vi "MDM_test.vi"() -> ()   [LabVIEW 2014]
uses:
  sub_VI/Control 1.ctl
  controls/thrust_control.ctl
  controls/diag.ctl
  <vilib>/Instr/_visa.llb/VISA Configure Serial Port (Instr).vi
  <vilib>/Utility/inputDevices.llb/joystickAcquire.vi
panel:
  in  "Calibrate Pressure":sgl=15.0 format="%_3f"
  in  "Calibrate Pressure":bool
  out "Pressure":sgl(knob) scale=-100.0..100.0
  out "diag":T1 {"calibrate pressure" format="%_6f"}
  out "axis info":T2
  out "button info":T3
  out "direction info":T4
  in  "index":u16
  in  "Address 2":u16
  in  "Forward":bool
  in  "Thrust":u16
  in  "VISA resource name 2":refnum<visa-resource-name>
  in  "Read Diag":bool
  in  "Thruster 1":T5 {"Thrust" scale=0.0..100.0}
  in  "baud rate (9600)":T6=19200
  in  "stop":bool
  in  "Address":u16
  in  "VISA resource name":refnum<visa-resource-name>="COM5"
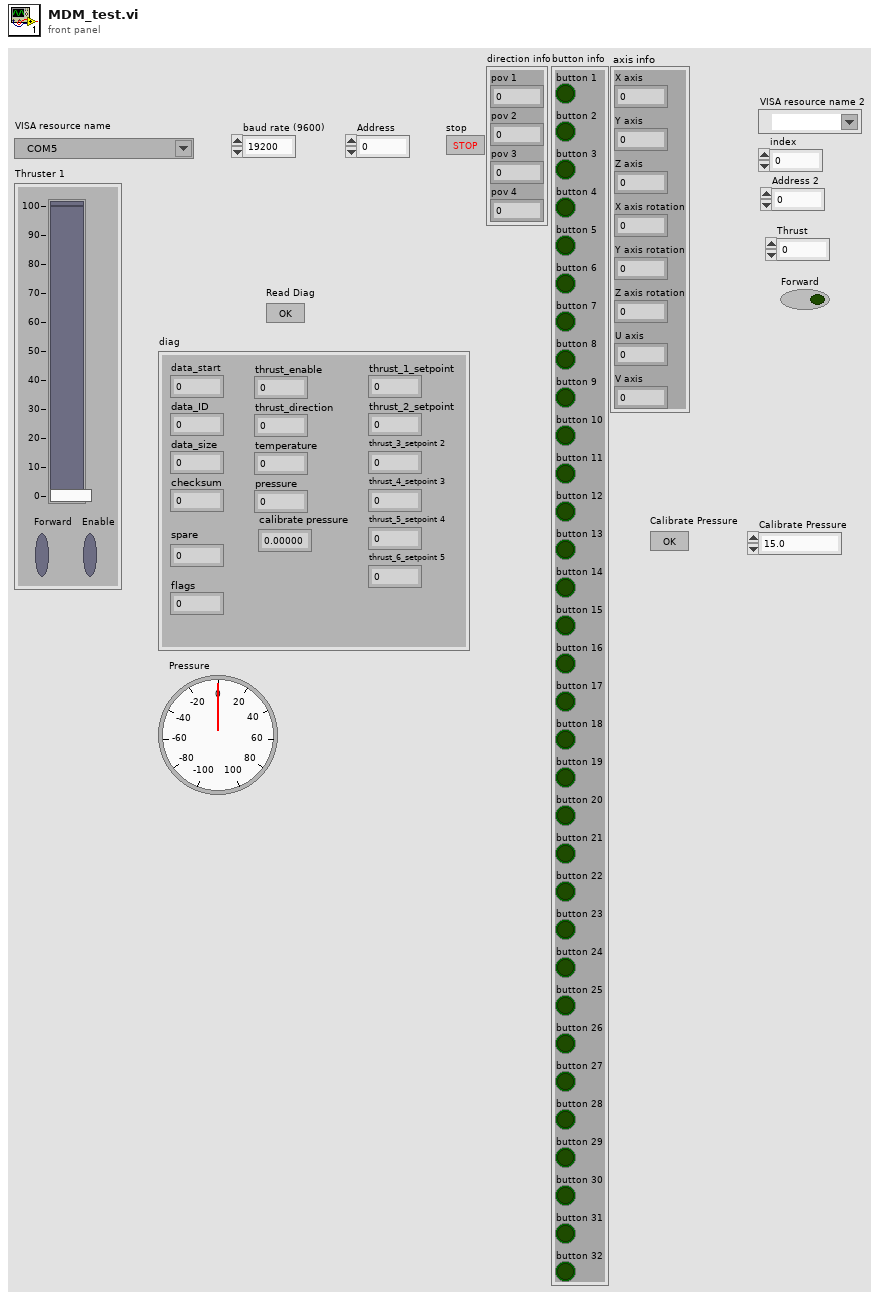
[diagram p1: front panel]
types:
  T1 = typedef "diag.ctl" = cluster{"data_start":u16, "data_ID":u16, "data_size":u16, "thrust_enable":u8, "thrust_direction":u8, "temperature":sgl, "pressure":sgl, "thrust_1_setpoint":u16, "thrust_2_setpoint":u16, "thrust_3_setpoint 2":u16, "thrust_4_setpoint 3":u16, "thrust_5_setpoint 4":u16, "thrust_6_setpoint 5":u16, "spare":u16, "flags":u16, "calibrate pressure":sgl, "checksum":u16}
  T2 = cluster{"X axis":i32, "Y axis":i32, "Z axis":i32, "X axis rotation":i32, "Y axis rotation":i32, "Z axis rotation":i32, "U axis":i32, "V axis":i32}
  T3 = cluster{"button 1":bool, "button 2":bool, "button 3":bool, "button 4":bool, "button 5":bool, "button 6":bool, "button 7":bool, "button 8":bool, "button 9":bool, "button 10":bool, "button 11":bool, "button 12":bool, "button 13":bool, "button 14":bool, "button 15":bool, "button 16":bool, "button 17":bool, "button 18":bool, "button 19":bool, "button 20":bool, "button 21":bool, "button 22":bool, "button 23":bool, "button 24":bool, "button 25":bool, "button 26":bool, "button 27":bool, "button 28":bool, "button 29":bool, "button 30":bool, "button 31":bool, "button 32":bool}
  T4 = cluster{"pov 1":i32, "pov 2":i32, "pov 3":i32, "pov 4":i32}
  T5 = typedef "thrust_control.ctl" = cluster{"Thrust":dbl, "Forward":bool, "Enable":bool}
  T6 = typedef "Control 1.ctl" = u32
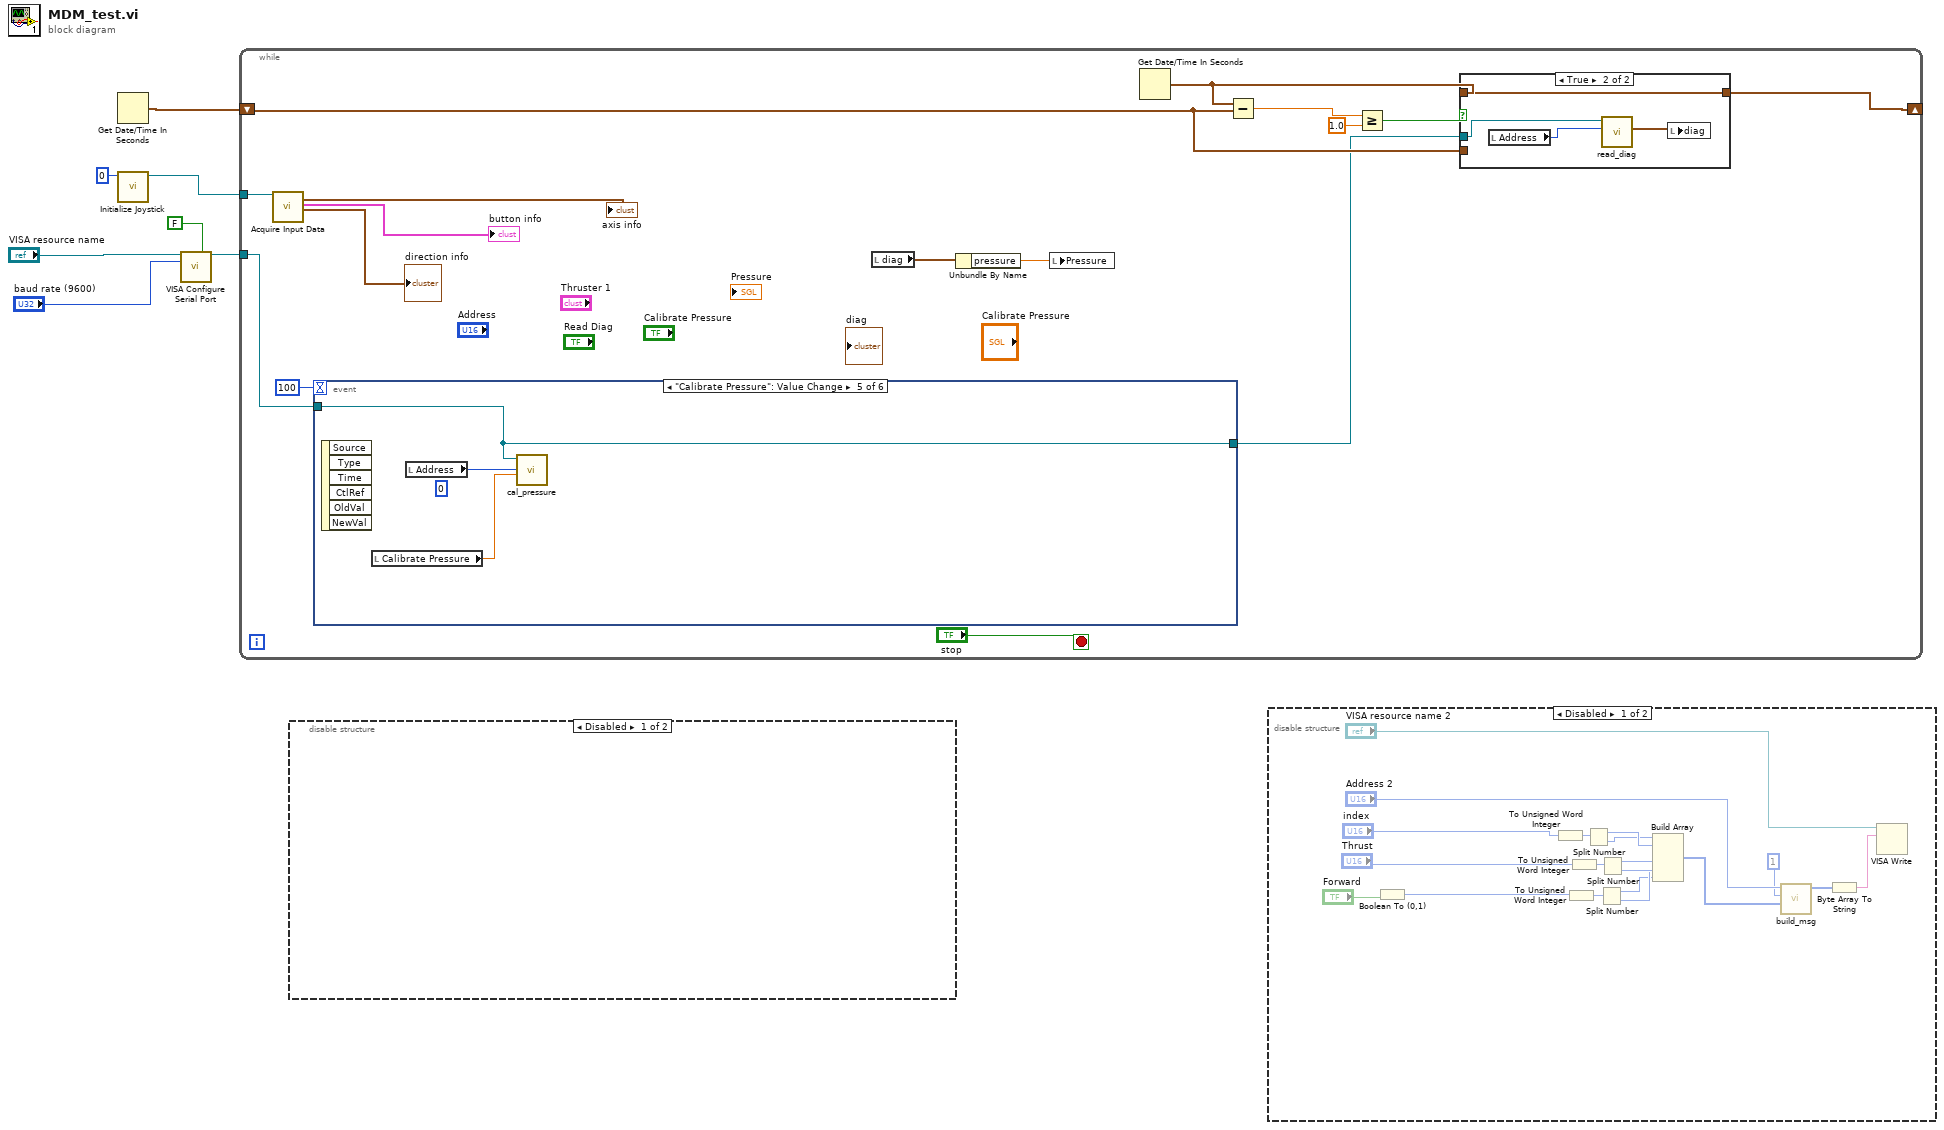
[diagram p0: block diagram]
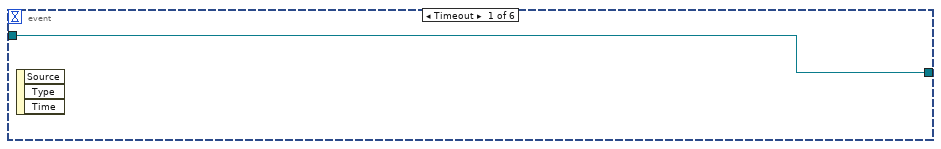
[diagram p5: hidden frame]
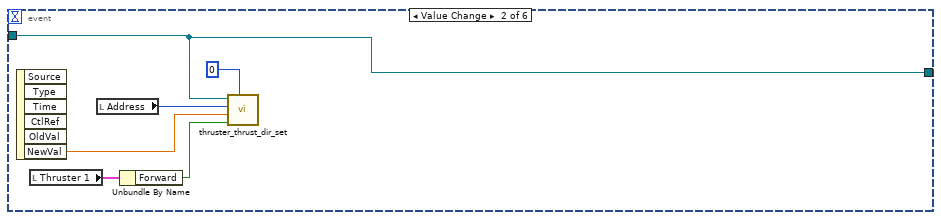
[diagram p6: hidden frame]
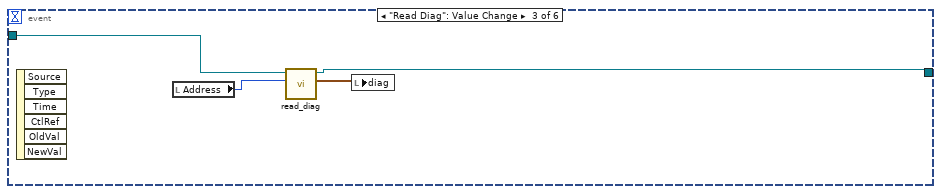
[diagram p7: hidden frame]
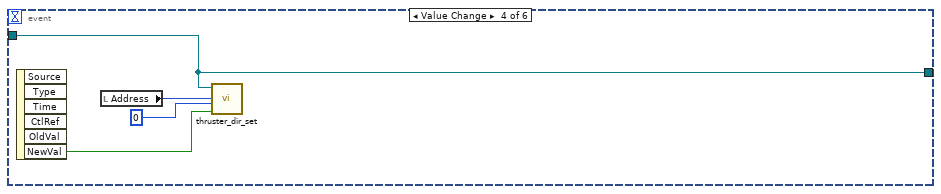
[diagram p8: hidden frame]
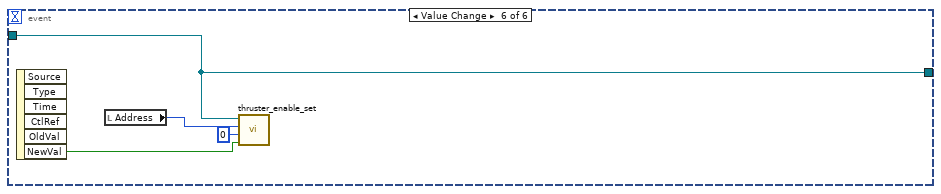
[diagram p9: hidden frame]
diagram:
  n1 = Get Date/Time In Seconds() -> (seconds since 1Jan1904=w1:timestamp)
  n2 = call <vilib>:"Initialize Joystick.vi"("device index"=0) -> ("device ID"=w3:refnum<k1>)  [unwired: 9 in, 1 out]
  n3 = call-poly "VISA Configure Serial Port"("VISA resource name"="VISA resource name", "Enable Termination\nChar (T)"=FALSE ("Enable Termination\nChar (T)"), "baud rate (9600)"="baud rate (9600)") -> ("VISA resource name out"=w7:refnum<visa-resource-name>)  [unwired: 11 in, 1 out]
  n4 = while {
    tunnel: w7 -> [w11]
    tunnel: w3 -> [w21]
    shift-right: [w12] -> _
    shift-left: w1 -> [w14]
    stop <- "stop" stop-if-true
    n5 = call-poly <vilib>:"Acquire Input Data.vi"("device ID"=w21) -> ("axis info"=→"axis info":T2, "button info"=→"button info":T3, "direction info"=→"direction info":T4)  [unwired: 14 in, 2 out]
    n6 = event shown="[4] \"Calibrate Pressure\": Value Change" {
      selector: _ -> [_ _ _ _ _ _]
      dyn-events: _ -> [_ _ _ _ _ _]
      timeout: 100 -> [_ _ _ _ _ _]
      tunnel: w11 -> [w29 w30 w39 w40 w45 w47]
      tunnel: [w29 w30 w36 w40 w45 w47] -> w10
      event Timeout {
        n7 = event-data() -> ()  [unwired: 1 in, 3 out]
      }
      event Value Change {
        n8 = event-data() -> ("NewVal"=w33:dbl)  [unwired: 1 in, 5 out]
        n9 = local read "Thruster 1"() -> (w32:T5)
        n10 = local read "Address"() -> (w35:u16)
        n11 = Unbundle By Name(w32) -> ("Forward"=w31:bool)
        n12 = call "thruster_thrust_dir_set.vi"("index"=u16 0, "Forward"=w31, "Thrust"=w33, "Address"=w35, "VISA resource name"=w30) -> ()  [unwired: 7 in]
      }
      event "Read Diag": Value Change {
        n13 = event-data() -> ()  [unwired: 1 in, 6 out]
        n14 = local read "Address"() -> (w38:u16)
        n15 = call "read_diag.vi"("Address"=w38, "VISA resource name"=w39) -> ("diag"=w37:T1, "VISA resource name out"=w36:refnum<visa-resource-name>)  [unwired: 7 in, 1 out]
        n16 = local write "diag"(w37) -> ()
      }
      event Value Change {
        n17 = event-data() -> ("NewVal"=w41:bool)  [unwired: 1 in, 5 out]
        n18 = local read "Address"() -> (w43:u16)
        n19 = call "thruster_dir_set.vi"("Forward"=w41, "index"=u16 0, "Address"=w43, "VISA resource name"=w40) -> ()  [unwired: 8 in]
      }
      event "Calibrate Pressure": Value Change {
        (unwired) u16 0 ("index")
        n20 = event-data() -> ()  [unwired: 1 in, 6 out]
        n21 = local read "Calibrate Pressure"() -> (w44:sgl)
        n22 = local read "Address"() -> (w46:u16)
        n23 = call "cal_pressure.vi"("calibration pressure"=w44, "Address"=w46, "VISA resource name"=w45) -> ()  [unwired: 9 in]
      }
      event Value Change {
        n24 = event-data() -> ("NewVal"=w48:bool)  [unwired: 1 in, 5 out]
        n25 = local read "Address"() -> (w50:u16)
        n26 = call "thruster_enable_set.vi"("enable"=w48, "index"=u16 0, "Address"=w50, "VISA resource name"=w47) -> ()  [unwired: 8 in]
      }
    }
    n27 = local read "diag"() -> (w9:T1)
    n28 = Unbundle By Name(w9) -> ("pressure"=w8:sgl)
    n29 = local write "Pressure"(w8) -> ()
    n30 = Get Date/Time In Seconds() -> (seconds since 1Jan1904=w13:timestamp)
    n31 = Subtract(x=w13, y=w14) -> (x-y=w17:dbl)
    n32 = Greater Or Equal?(x=w17, y=1.0) -> (x >= y?=w15:bool)
    n33 = case shown="True" w15 {
      tunnel: w14 -> [w24 _]
      tunnel: w13 -> [_ w28]
      tunnel: [w24 w28] -> w12
      tunnel: w10 -> [_ w25]
      frame False {
      }
      frame True {
        n34 = local read "Address"() -> (w26:u16)
        n35 = call "read_diag.vi"("Address"=w26, "VISA resource name"=w25) -> ("diag"=w27:T1)  [unwired: 7 in, 2 out]
        n36 = local write "diag"(w27) -> ()
      }
    }
  }
  n37 = disable-structure shown="Disabled" {
    frame Disabled {
    }
    frame Enabled {
    }
  }
  n38 = disable-structure shown="Disabled" {
    frame Disabled {
      n39 = Boolean To (0,1)(Boolean="Forward") -> (0, 1=w63:i16)
      n40 = To Unsigned Word Integer(number="index") -> (unsigned 16bit integer=w66:u16)
      n41 = To Unsigned Word Integer(number=w63) -> (unsigned 16bit integer=w57:u16)
      n42 = To Unsigned Word Integer(number="Thrust") -> (unsigned 16bit integer=w51:u16)
      n43 = Split Number(x=w66) -> (hi(x)=w68:u8, lo(x)=w67:u8)
      n44 = Split Number(x=w57) -> (hi(x)=w53:u8, lo(x)=w54:u8)
      n45 = Split Number(x=w51) -> (hi(x)=w55:u8, lo(x)=w56:u8)
      n46 = Build Array(w67, w68, w56, w55, w54, w53) -> (w52:u8[])
      n47 = call "build_msg.vi"("data"=w52, "ID"=u16 1, "Address"="Address 2") -> ("msg"=w59:u8[])  [unwired: 8 in]
      n48 = Byte Array To String(unsigned byte array=w59) -> (string=w60:string)
      n49 = VISA Write(VISA resource name="VISA resource name 2", write buffer=w60) -> ()  [unwired: 1 in, 3 out]
    }
    frame Enabled {
    }
  }
